vi "setValvesArduinoNew.vi"(11 "valve data":bool[](array[boolean])=[FALSE, FALSE, FALSE, FALSE, FALSE, FALSE, FALSE, FALSE]) -> ()   [LabVIEW 2012]
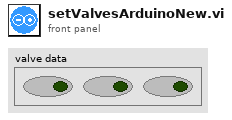
[diagram p1: front panel]
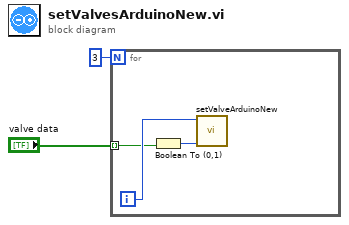
[diagram p0: block diagram]
diagram:
  n1 = for {
    N: 3 -> [_]
    tunnel: "valve data" -> [w3] mode=indexing
    i -> [w5]
    n2 = Boolean To (0,1)(Boolean=w3) -> (0, 1=w4:i16)
    n3 = call "setValveArduinoNew.vi"("value"=w4, "valve id"=w5) -> ()  [unwired: 10 in]
  }
